vi "LVProjectShortcut_Item_OnCommand.vi"(10 "Command ID":string, 11 "Object":T1) -> ()   [LabVIEW 2017]
uses:
  <resource>/Framework/Providers/API/ItemRef.ctl
panel:
  out "error out":errorcluster
  in  "error in":errorcluster
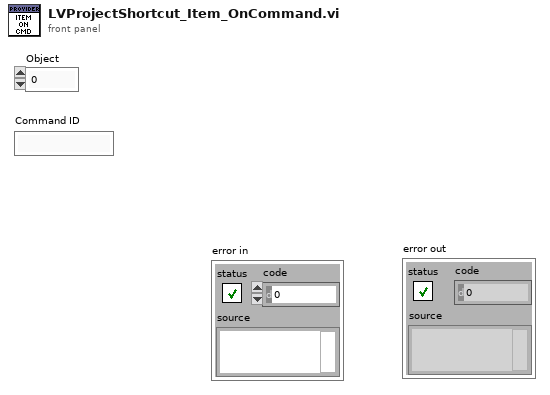
[diagram p1: front panel]
types:
  T1 = typedef "ItemRef.ctl" = u64
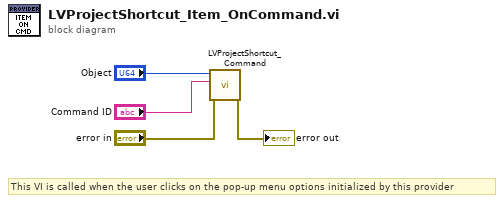
[diagram p0: block diagram]
diagram:
  # "This VI is called when the user clicks on the pop-up menu options initialized by this provider"
  n1 = call <resource>:"LVProjectShortcut_Command.vi"("error in"="error in", "Command"="Command ID", "Object"="Object") -> ("error out"=→"error out":errorcluster)  [unwired: 8 in]
